vi "Status Log FGV.vi"(7 "Action":T1=enum."Show Status File", 8 "error in":errorcluster, 10 "Status":string) -> (0 "error out":errorcluster)   [LabVIEW 2015]
doc: "FGV for managign starus log file"
uses:
  Status Log.ctl
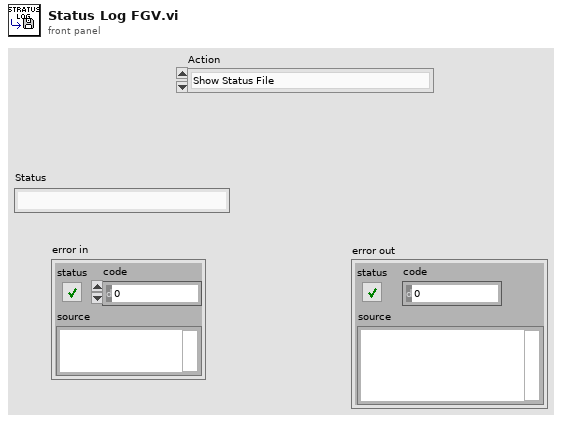
[diagram p1: front panel]
types:
  T1 = typedef "Status Log.ctl" = enum16{"Close file", "Open Status file", "Add Status", "Show Status File"}
  T2 = enum16{"open", "replace", "create", "open or create", "replace or create", "replace or create with confirmation"}
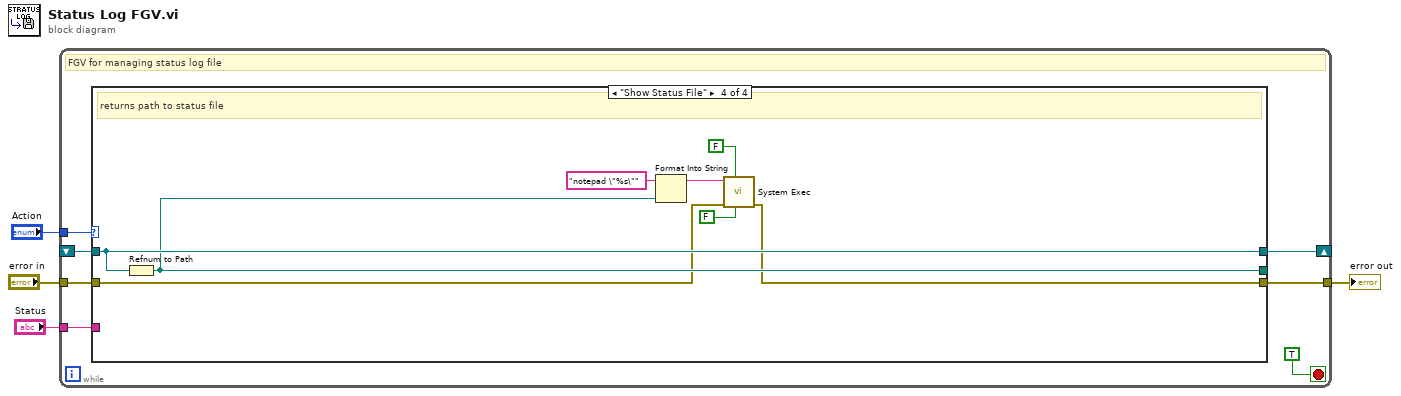
[diagram p0: block diagram]
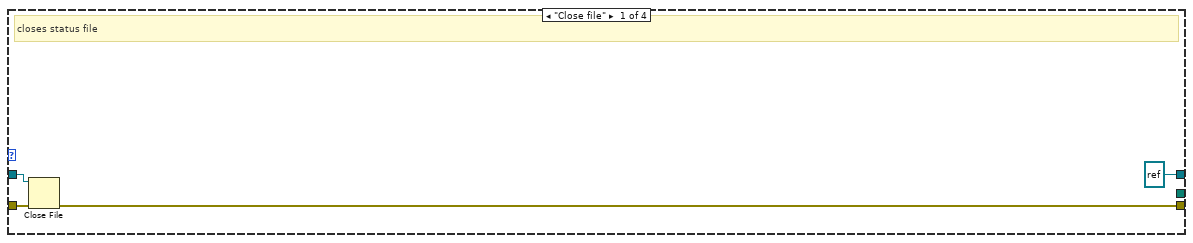
[diagram p2: hidden frame]
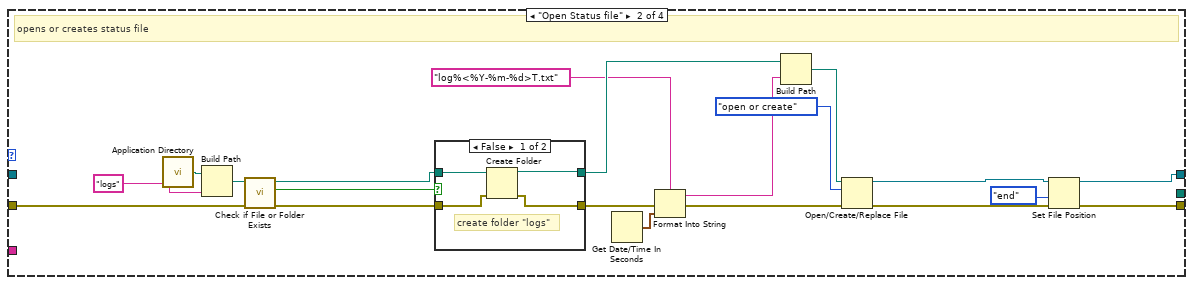
[diagram p3: hidden frame]
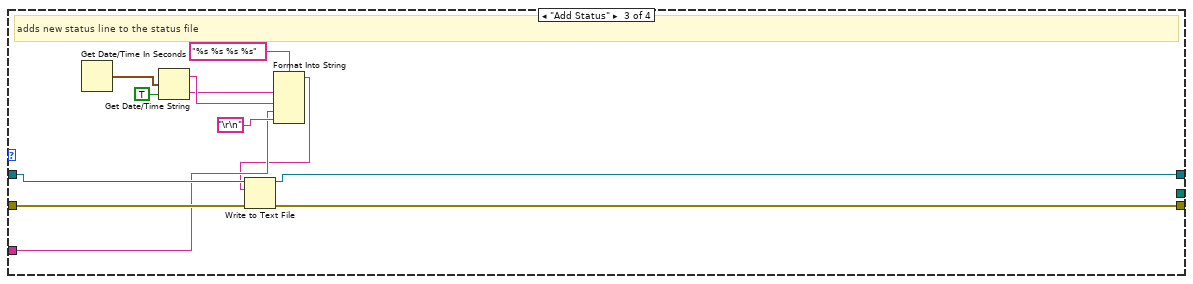
[diagram p5: hidden frame]
diagram:
  n1 = while {
    tunnel: "Action" -> [w10]
    tunnel: "Status" -> [w9]
    tunnel: [w8] -> w2
    tunnel: "error in" -> [w7]
    shift-right: [w5] -> _
    shift-left: _ -> [w6]
    stop <- TRUE stop-if-true
    # "FGV for managing status log file"
    n2 = case shown="\"Show Status File\"" w10 {
      tunnel: w9 -> [_ _ w43 _]
      tunnel: [w14 w27 w53 w57] -> w8
      tunnel: w7 -> [w15 w20 w50 w58]
      tunnel: [refnum<file> refnum ("refnum out") w26 w52 w61] -> w5
      tunnel: w6 -> [w13 _ w51 w61]
      tunnel: [_ _ _ w59] -> _
      frame "Close file" {
        # "closes status file"
        n3 = Close File(refnum=w13, error in=w15) -> (error out=w14:errorcluster)  [unwired: 1 out]
      }
      frame "Open Status file" {
        # "opens or creates status file"
        n4 = call <vilib>:"Application Directory.vi"() -> ("Application Directory"=w35:path)
        n5 = Build Path(base path=w35, name or relative path="logs") -> (appended path=w25:path)
        n6 = call <vilib>:"Check if File or Folder Exists.vi"("error in (no error)"=w20, "path"=w25) -> ("error out"=w21:errorcluster, "file or folder exists?"=w24:bool, "dup path"=w23:path)  [unwired: 7 in]
        n7 = case shown="False" w24 {
          tunnel: w23 -> [w39 w41]
          tunnel: [w38 w41] -> w22
          tunnel: w21 -> [w37 w40]
          tunnel: [w36 w40] -> w19
          frame False {
            # "create folder \"logs\""
            n8 = Create Folder(path (use dialog)=w39, error in=w37) -> (created path=w38:path, error out=w36:errorcluster)  [unwired: 1 in, 1 out]
          }
          frame True {
          }
        }
        n9 = Get Date/Time In Seconds() -> (seconds since 1Jan1904=w34:timestamp)
        n10 = Format Into String "Format Into String"(format string="log%<%Y-%m-%d>T.txt", error in=w19, w34) -> (resulting string=w32:string, error out=w33:errorcluster)  [unwired: 1 in]
        n11 = Build Path(base path=w22, name or relative path=w32) -> (appended path=w31:path)
        n12 = Open/Create/Replace File(file path (use dialog)=w31, error in=w33, operation (0:open)=T2."open or create") -> (refnum out=w28:refnum<file>, error out=w29:errorcluster)  [unwired: 3 in, 1 out]
        n13 = Set File Position(refnum=w28, from (0:start)=enum16{"start", "end", "current"}."end", error in=w29) -> (refnum out=w26:refnum<file>, error out=w27:errorcluster)  [unwired: 1 in]
      }
      frame "Add Status" {
        # "adds new status line to the status file"
        n14 = Get Date/Time In Seconds() -> (seconds since 1Jan1904=w48:timestamp)
        n15 = Get Date/Time String(seconds (now)=w48, want seconds? (F)=TRUE) -> (date string=w47:string, time string=w46:string)  [unwired: 1 in]
        n16 = Format Into String(format string="%s %s %s %s", w46, w47, w43, "\r\n") -> (resulting string=w42:string)  [unwired: 2 in, 1 out]
        n17 = Write to Text File(file (use dialog)=w51, text=w42, error in=w50) -> (refnum out=w52:refnum<file>, error out=w53:errorcluster)  [unwired: 1 in, 1 out]
      }
      frame "Show Status File" {
        # "returns path to status file"
        n18 = Refnum to Path(1:w61) -> (0:w59:path)
        n19 = Format Into String(initial string="notepad \"%s\"", w59) -> (resulting string=w60:string)  [unwired: 2 in, 1 out]
        n20 = call <vilib>:"System Exec.vi"("run minimized? (F)"=FALSE, "wait until completion? (T)"=FALSE, "error in (no error)"=w58, "command line"=w60) -> ("error out"=w57:errorcluster)  [unwired: 4 in, 3 out]
      }
    }
  }
  "error out" <- w2
